vi "PH_gentec_Powermeter.set current Sets to GUI.vi"(0 "i ref in":refnum<vi>, 5 "error in":errorcluster) -> (14 "i ref out":refnum<vi>, 19 "error out":errorcluster)   [LabVIEW 2014, in "PH_gentec_Powermeter.lvlib"]
doc: "This VI indicates the wanted Settings at the GUI element."
uses:
  PH_gentec_Powermeter.lvlib
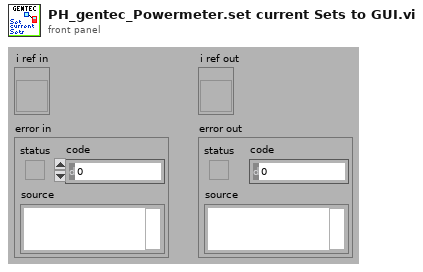
[diagram p1: front panel]
types:
  T1 = typedef "PH_gentec_Powermeter.lvlib/PH_gentec_Powermeter.i attribute.ctl" = cluster{"GUI References":cluster{"delete":refnum<vi>, "start stop Statistics":refnum<vi>, "Statistic Data":refnum<vi>, "Configuration Values":refnum<vi>, "Set Zero":refnum<vi>, "Data Sampling Settings":refnum<vi>, "Wanted Sets":refnum<vi>, "Current Sets":refnum<vi>}, "Start Stop Statistics":bool, "Wanted Sets":T2, "Current Sets":T2}
  T2 = typedef "PH_gentec_Powermeter.lvlib/PH_gentec_Powermeter.Sets.ctl" = cluster{"Data Sampling Settings":T3, "Set Zero":bool}
  T3 = typedef "gentec-SOLO-PE - Driver.lvlib/gentec-SOLO-PE.Data Sampling Settings.ctl" = cluster{"Sample Rate":u32, "Sample Rate Unit":u32, "Sample Period":u32, "Sample Period Unit":u32, "Total Duration":u32, "Total Duration Unit":u32, "Time Stamp":u32}
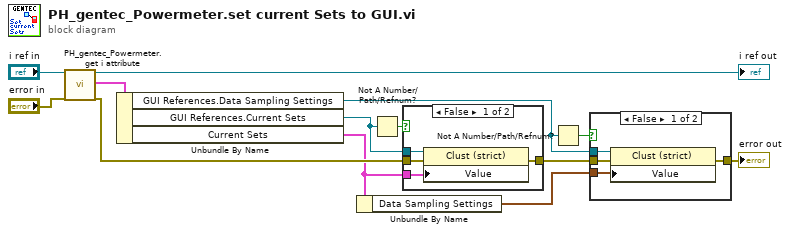
[diagram p0: block diagram]
diagram:
  n1 = call "PH_gentec_Powermeter.get i attribute.vi"("i ref in"="i ref in", "error in (no error)"="error in") -> ("i ref out"=→"i ref out":refnum<vi>, "i attribute"=w12:T1, "error out"=w11:errorcluster)  [unwired: 15 in]
  n2 = Unbundle By Name(w12) -> ("GUI References.Data Sampling Settings"=w3:refnum<vi>, "GUI References.Current Sets"=w9:refnum<vi>, "Current Sets"=w10:T2)
  n3 = Unbundle By Name(w10) -> ("Data Sampling Settings"=w2:T3)
  n4 = Not A Number/Path/Refnum?(number/path/refnum=w9) -> (NaN/Path/Refnum?=w13:bool)
  n5 = case shown="False" w13 {
    tunnel: [w16 w18] -> w1
    tunnel: w9 -> [w15 _]
    tunnel: w11 -> [w17 w18]
    tunnel: w10 -> [w14 _]
    frame False {
      n6 = property class="Clust (strict)"(reference=w15, error in=w17, "Value"=w14) -> (error out=w16:errorcluster)  [unwired: 1 out]
    }
    frame True {
    }
  }
  n7 = Not A Number/Path/Refnum?(number/path/refnum=w3) -> (NaN/Path/Refnum?=w5:bool)
  n8 = case shown="False" w5 {
    tunnel: [w19 w23] -> w4
    tunnel: w3 -> [w22 _]
    tunnel: w1 -> [w21 w23]
    tunnel: w2 -> [w20 _]
    frame False {
      n9 = property class="Clust (strict)"(reference=w22, error in=w21, "Value"=w20) -> (error out=w19:errorcluster)  [unwired: 1 out]
    }
    frame True {
    }
  }
  "error out" <- w4
